vi "CW graph.vi"() -> ()   [LabVIEW 2023]
uses:
  <vilib>/Utility/file.llb/Read Delimited Spreadsheet (DBL).vi
panel:
  out "recovery":dbl
  out "stage4":dbl
  out "stage3":dbl
  out "stage2":dbl
  out "stage1":dbl
  out "baseline":dbl
  out "Waveform Graph":dbl[](graph)
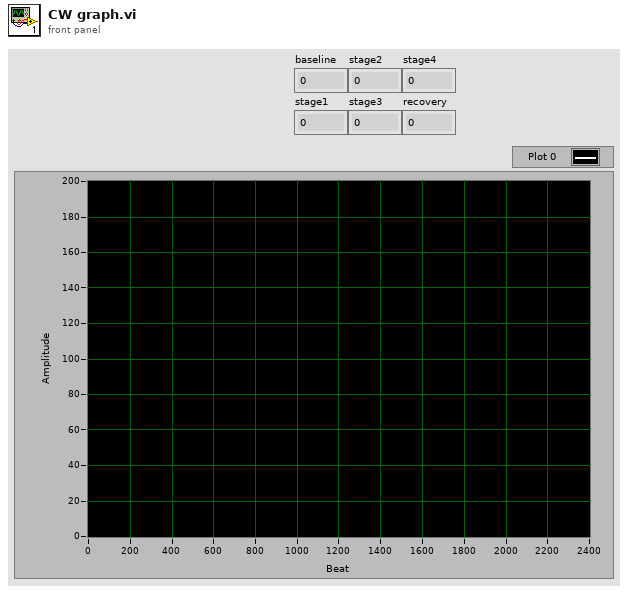
[diagram p1: front panel]
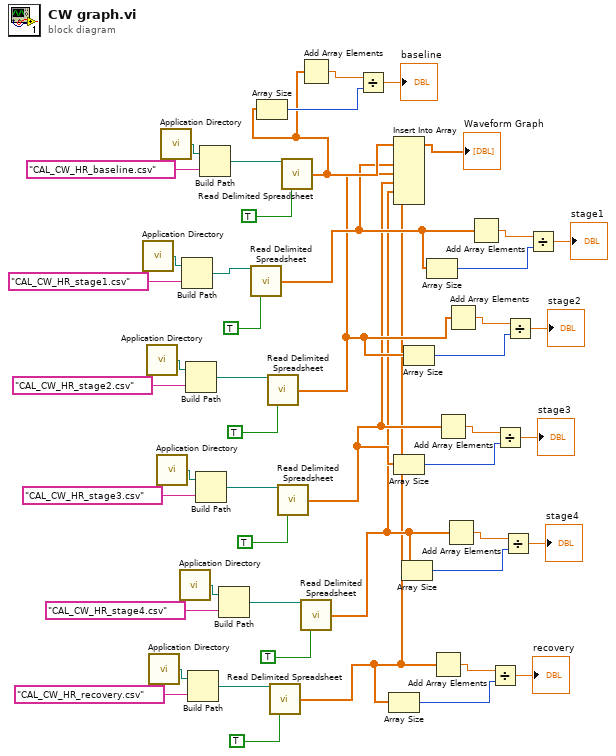
[diagram p0: block diagram]
diagram:
  n1 = call <vilib>:"Application Directory.vi"() -> ("Application Directory"=w45:path)
  n2 = call <vilib>:"Application Directory.vi"() -> ("Application Directory"=w41:path)
  n3 = call <vilib>:"Application Directory.vi"() -> ("Application Directory"=w29:path)
  n4 = call <vilib>:"Application Directory.vi"() -> ("Application Directory"=w37:path)
  n5 = call <vilib>:"Application Directory.vi"() -> ("Application Directory"=w49:path)
  n6 = call <vilib>:"Application Directory.vi"() -> ("Application Directory"=w33:path)
  n7 = Build Path(base path=w45, name or relative path="CAL_CW_HR_stage1.csv") -> (appended path=w42:path)
  n8 = Build Path(base path=w41, name or relative path="CAL_CW_HR_stage2.csv") -> (appended path=w38:path)
  n9 = Build Path(base path=w29, name or relative path="CAL_CW_HR_recovery.csv") -> (appended path=w26:path)
  n10 = Build Path(base path=w37, name or relative path="CAL_CW_HR_stage3.csv") -> (appended path=w34:path)
  n11 = Build Path(base path=w49, name or relative path="CAL_CW_HR_baseline.csv") -> (appended path=w46:path)
  n12 = Build Path(base path=w33, name or relative path="CAL_CW_HR_stage4.csv") -> (appended path=w30:path)
  n13 = call-poly <vilib>:"Read Delimited Spreadsheet.vi"("file path (dialog if empty)"=w42, "transpose? (F)"=TRUE) -> ("first row"=w17:dbl[])  [unwired: 8 in, 5 out]
  n14 = call-poly <vilib>:"Read Delimited Spreadsheet.vi"("file path (dialog if empty)"=w38, "transpose? (F)"=TRUE) -> ("first row"=w13:dbl[])  [unwired: 8 in, 5 out]
  n15 = call-poly <vilib>:"Read Delimited Spreadsheet.vi"("file path (dialog if empty)"=w26, "transpose? (F)"=TRUE) -> ("first row"=w1:dbl[])  [unwired: 8 in, 5 out]
  n16 = call-poly <vilib>:"Read Delimited Spreadsheet.vi"("file path (dialog if empty)"=w34, "transpose? (F)"=TRUE) -> ("first row"=w9:dbl[])  [unwired: 8 in, 5 out]
  n17 = call-poly <vilib>:"Read Delimited Spreadsheet.vi"("file path (dialog if empty)"=w46, "transpose? (F)"=TRUE) -> ("first row"=w23:dbl[])  [unwired: 8 in, 5 out]
  n18 = Array Size(array=w23) -> (size(s)=w24:i32)
  n19 = Add Array Elements(numeric array=w23) -> (sum=w22:dbl)
  n20 = call-poly <vilib>:"Read Delimited Spreadsheet.vi"("file path (dialog if empty)"=w30, "transpose? (F)"=TRUE) -> ("first row"=w5:dbl[])  [unwired: 8 in, 5 out]
  n21 = Divide(x=w22, y=w24) -> (x/y=→"baseline":dbl)
  n22 = Array Size(array=w1) -> (size(s)=w4:i32)
  n23 = Insert Into Array(array=w23, new element #1=w17, new element #2=w13, new element #3=w9, new element #4=w5, new element #5=w1) -> (→"Waveform Graph":dbl[])  [unwired: 1 in]
  n24 = Array Size(array=w9) -> (size(s)=w12:i32)
  n25 = Array Size(array=w5) -> (size(s)=w8:i32)
  n26 = Array Size(array=w13) -> (size(s)=w16:i32)
  n27 = Array Size(array=w17) -> (size(s)=w20:i32)
  n28 = Add Array Elements(numeric array=w1) -> (sum=w3:dbl)
  n29 = Add Array Elements(numeric array=w9) -> (sum=w11:dbl)
  n30 = Add Array Elements(numeric array=w5) -> (sum=w7:dbl)
  n31 = Add Array Elements(numeric array=w13) -> (sum=w15:dbl)
  n32 = Add Array Elements(numeric array=w17) -> (sum=w19:dbl)
  n33 = Divide(x=w3, y=w4) -> (x/y=→"recovery":dbl)
  n34 = Divide(x=w11, y=w12) -> (x/y=→"stage3":dbl)
  n35 = Divide(x=w7, y=w8) -> (x/y=→"stage4":dbl)
  n36 = Divide(x=w15, y=w16) -> (x/y=→"stage2":dbl)
  n37 = Divide(x=w19, y=w20) -> (x/y=→"stage1":dbl)
